vi "bt-init_com.vi"(6 "timeout (10sec)":u32=10000, 7 "End Write on Termination Character?":bool, 8 "error in (no error)":errorcluster, 9 "VISA buffer":i32, 10 "baud rate":u32, 11 "VISA resource name":refnum<visa-resource-name>="COM13") -> (0 "error out":errorcluster)   [LabVIEW 2023, in "bt-interface.lvlib"]
uses:
  bt-interface.lvlib
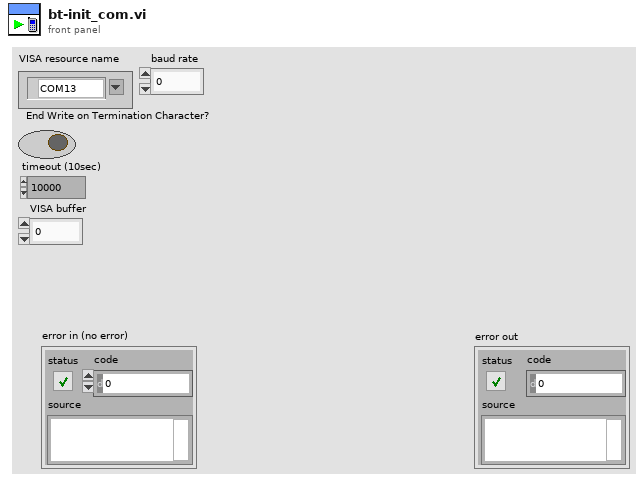
[diagram p1: front panel]
types:
  T1 = enum16{"init", "broadcast_data", "receive_data", "close", "clear_visa"}
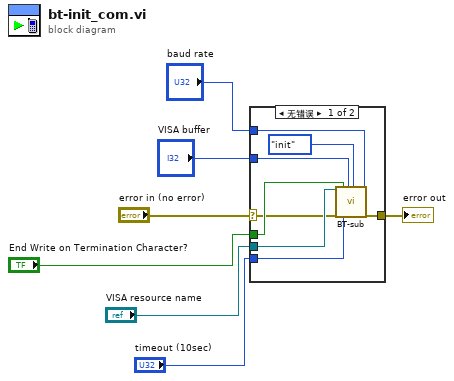
[diagram p0: block diagram]
diagram:
  n1 = case shown="无错误" "error in (no error)" {
    selector: "error in (no error)" -> [w9 w16]
    tunnel: [w8 w16] -> w6
    tunnel: "VISA resource name" -> [w10 _]
    tunnel: "End Write on Termination Character?" -> [w12 _]
    tunnel: "timeout (10sec)" -> [w11 _]
    tunnel: "baud rate" -> [w15 _]
    tunnel: "VISA buffer" -> [w13 _]
    frame No Error {
      n2 = call "BT-sub.vi"("VISA resource name"=w10, "error in (no error)"=w9, "End Write on Termination Character?"=w12, "timeout (10sec)"=w11, "VISA buffer"=w13, "mode"=T1."init", "baud rate"=w15) -> ("error IO"=w8:errorcluster)  [unwired: 10 in, 2 out]
    }
    frame Error {
    }
  }
  "error out" <- w6
